vi "GetColor.vi"(1 "输入":u32[][](array[numeric])) -> (0 "颜色":u32)   [LabVIEW 2016]
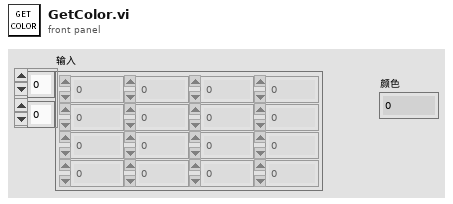
[diagram p1: front panel]
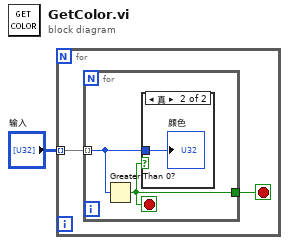
[diagram p0: block diagram]
diagram:
  n1 = for {
    tunnel: "输入" -> [w3] mode=indexing
    stop <- w2 stop-if-true
    n2 = for {
      tunnel: w3 -> [w5] mode=indexing
      tunnel: [w4] -> w2
      stop <- w4 stop-if-true
      n3 = Greater Than 0?(x=w5) -> (x > 0?=w4:bool)
      n4 = case shown="真" w4 {
        tunnel: w5 -> [_ w6]
        frame False {
        }
        frame True {
          "颜色" <- w6
        }
      }
    }
  }
